vi "XY_Stage_Movement.vi"(10 "Y Input":dbl, 11 "X Input":dbl) -> (2 "Current Y Position":sgl, 3 "Current X Position":sgl)   [LabVIEW 2013]
panel:
  out "Original Y Position":sgl
  out "Original X Position":sgl
  in  "Y Stage Serial":i32
  in  "X Stage Serial":i32
  in  "Y Stage Motor":refnum<k7>(container)
  in  "X Stage motor":refnum<k7>(container)
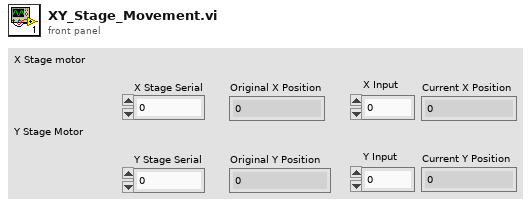
[diagram p1: front panel]
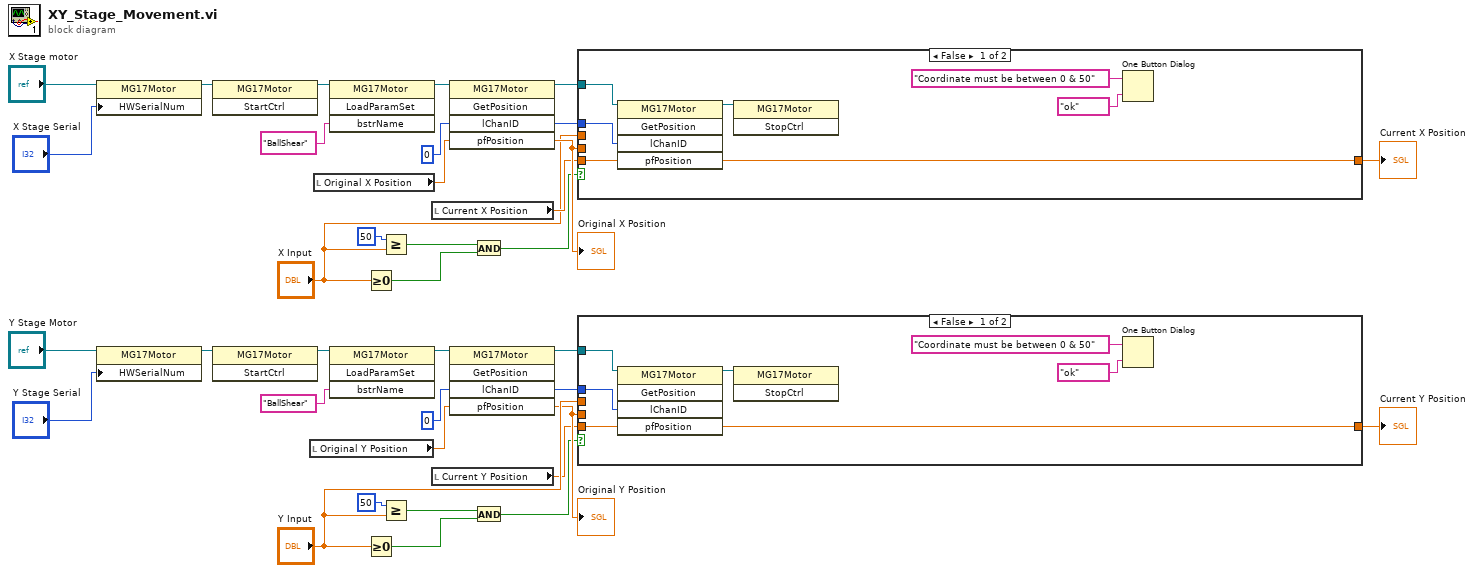
[diagram p0: block diagram]
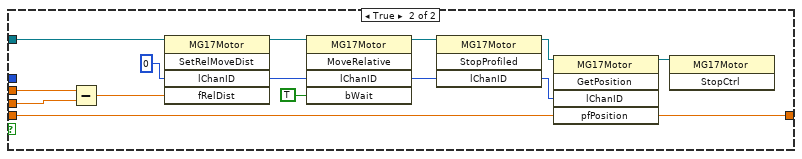
[diagram p2: hidden frame]
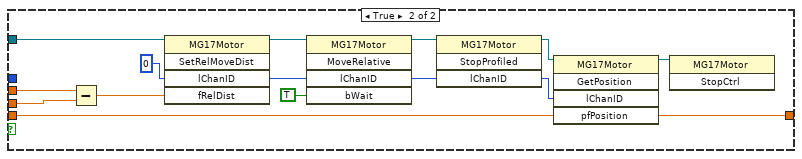
[diagram p3: hidden frame]
diagram:
  n1 = property class="MG17Motor"(reference="X Stage motor", "HWSerialNum"="X Stage Serial") -> (reference out=w31:refnum<k7>)  [unwired: 1 in, 1 out]
  n2 = property class="MG17Motor"(reference="Y Stage Motor", "HWSerialNum"="Y Stage Serial") -> (reference out=w32:refnum<k7>)  [unwired: 1 in, 1 out]
  n3 = invoke class="MG17Motor" method="StartCtrl"(reference=w31) -> (reference out=w13:refnum<k7>)  [unwired: 2 in, 2 out]
  n4 = invoke class="MG17Motor" method="StartCtrl"(reference=w32) -> (reference out=w10:refnum<k7>)  [unwired: 2 in, 2 out]
  n5 = local read "Original Y Position"() -> (w21:sgl)
  n6 = local read "Original X Position"() -> (w29:sgl)
  n7 = invoke class="MG17Motor" method="LoadParamSet"(reference=w13, "bstrName"="BallShear") -> (reference out=w12:refnum<k7>)  [unwired: 2 in, 3 out]
  n8 = invoke class="MG17Motor" method="LoadParamSet"(reference=w10, "bstrName"="BallShear") -> (reference out=w9:refnum<k7>)  [unwired: 2 in, 3 out]
  n9 = Greater Or Equal To 0?(x="X Input") -> (x >= 0?=w28:bool)
  n10 = Greater Or Equal To 0?(x="Y Input") -> (x >= 0?=w20:bool)
  n11 = Greater Or Equal?(x=50, y="X Input") -> (x >= y?=w27:bool)
  n12 = Greater Or Equal?(x=50, y="Y Input") -> (x >= y?=w19:bool)
  n13 = local read "Current X Position"() -> (w7:sgl)
  n14 = local read "Current Y Position"() -> (w5:sgl)
  n15 = invoke class="MG17Motor" method="GetPosition"(reference=w12, "lChanID"=0, "pfPosition"=w29) -> (reference out=w23:refnum<k7>, "lChanID"=w2:i32, "pfPosition"=w25:sgl)  [unwired: 2 in, 2 out]
  "Original X Position" <- w25
  n16 = invoke class="MG17Motor" method="GetPosition"(reference=w9, "lChanID"=0, "pfPosition"=w21) -> (reference out=w15:refnum<k7>, "lChanID"=w3:i32, "pfPosition"=w16:sgl)  [unwired: 2 in, 2 out]
  "Original Y Position" <- w16
  n17 = And(x=w27, y=w28) -> (x .and. y?=w24:bool)
  n18 = And(x=w19, y=w20) -> (x .and. y?=w8:bool)
  n19 = case shown="False" w24 {
    tunnel: "X Input" -> [_ w50]
    tunnel: w25 -> [_ w49]
    tunnel: w23 -> [w41 w51]
    tunnel: w7 -> [w39 w46]
    tunnel: [w38 w45] -> w6
    tunnel: w2 -> [w37 _]
    frame False {
      n20 = invoke class="MG17Motor" method="GetPosition"(reference=w41, "lChanID"=w37, "pfPosition"=w39) -> (reference out=w40:refnum<k7>, "pfPosition"=w38:sgl)  [unwired: 2 in, 3 out]
      n21 = invoke class="MG17Motor" method="StopCtrl"(reference=w40) -> ()  [unwired: 2 in, 3 out]
      n22 = One Button Dialog(message="Coordinate must be between 0 & 50", button name ("OK")="ok") -> ()  [unwired: 1 out]
    }
    frame True {
      n23 = Subtract(x=w50, y=w49) -> (x-y=w52:dbl)
      n24 = invoke class="MG17Motor" method="SetRelMoveDist"(reference=w51, "lChanID"=0, "fRelDist"=w52) -> (reference out=w55:refnum<k7>, "lChanID"=w56:i32)  [unwired: 2 in, 3 out]
      n25 = invoke class="MG17Motor" method="MoveRelative"(reference=w55, "lChanID"=w56, "bWait"=TRUE) -> (reference out=w57:refnum<k7>, "lChanID"=w58:i32)  [unwired: 2 in, 3 out]
      n26 = invoke class="MG17Motor" method="StopProfiled"(reference=w57, "lChanID"=w58) -> (reference out=w48:refnum<k7>, "lChanID"=w44:i32)  [unwired: 2 in, 2 out]
      n27 = invoke class="MG17Motor" method="GetPosition"(reference=w48, "lChanID"=w44, "pfPosition"=w46) -> (reference out=w47:refnum<k7>, "pfPosition"=w45:sgl)  [unwired: 2 in, 3 out]
      n28 = invoke class="MG17Motor" method="StopCtrl"(reference=w47) -> ()  [unwired: 2 in, 3 out]
    }
  }
  "Current X Position" <- w6
  n29 = case shown="False" w8 {
    tunnel: "Y Input" -> [_ w71]
    tunnel: w16 -> [_ w72]
    tunnel: w15 -> [w65 w73]
    tunnel: w5 -> [w61 w67]
    tunnel: [w60 w66] -> w4
    tunnel: w3 -> [w59 _]
    frame False {
      n30 = invoke class="MG17Motor" method="GetPosition"(reference=w65, "lChanID"=w59, "pfPosition"=w61) -> (reference out=w62:refnum<k7>, "pfPosition"=w60:sgl)  [unwired: 2 in, 3 out]
      n31 = invoke class="MG17Motor" method="StopCtrl"(reference=w62) -> ()  [unwired: 2 in, 3 out]
      n32 = One Button Dialog(message="Coordinate must be between 0 & 50", button name ("OK")="ok") -> ()  [unwired: 1 out]
    }
    frame True {
      n33 = Subtract(x=w71, y=w72) -> (x-y=w74:dbl)
      n34 = invoke class="MG17Motor" method="SetRelMoveDist"(reference=w73, "lChanID"=0, "fRelDist"=w74) -> (reference out=w77:refnum<k7>, "lChanID"=w78:i32)  [unwired: 2 in, 3 out]
      n35 = invoke class="MG17Motor" method="MoveRelative"(reference=w77, "lChanID"=w78, "bWait"=TRUE) -> (reference out=w79:refnum<k7>, "lChanID"=w80:i32)  [unwired: 2 in, 3 out]
      n36 = invoke class="MG17Motor" method="StopProfiled"(reference=w79, "lChanID"=w80) -> (reference out=w70:refnum<k7>, "lChanID"=w68:i32)  [unwired: 2 in, 2 out]
      n37 = invoke class="MG17Motor" method="GetPosition"(reference=w70, "lChanID"=w68, "pfPosition"=w67) -> (reference out=w69:refnum<k7>, "pfPosition"=w66:sgl)  [unwired: 2 in, 3 out]
      n38 = invoke class="MG17Motor" method="StopCtrl"(reference=w69) -> ()  [unwired: 2 in, 3 out]
    }
  }
  "Current Y Position" <- w4
